vi "Sample Rate Read.vi"(4 "error in (no error)":errorcluster, 6 "Container State":T2, 7 "Display State In":T1) -> (0 "error out":errorcluster, 2 "Value":dbl, 3 "Display State Out":T1)   [LabVIEW 2017, in "Test Signal Configuration.xctl"]
uses:
  <vilib>/addons/_XControls/Function Generator Configuration/Test Signal Configuration.xctl
  <vilib>/_xctls/Container State.ctl
  <vilib>/addons/_XControls/Function Generator Configuration/Controls/State.ctl
  <vilib>/_xctls/XControlSupport.lvlib
panel:
  # "Replace the Value Indicator below with an Indicator of desired type.\nDo not remove this Indicator or the others from the connector pane. \nDo not change the connector pane pattern.\nThe Value Indicator should always be the second terminal from top on the output side in the connector pane."
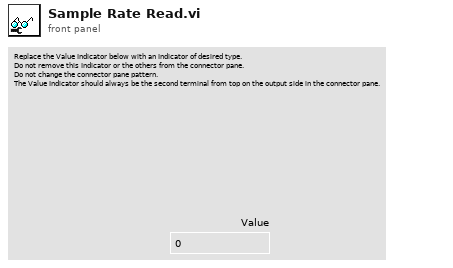
[diagram p1: front panel]
types:
  T1 = typedef "Test Signal Configuration.xctl/State.ctl" = cluster{"Attributes":variant}
  T2 = typedef "XControlSupport.lvlib/Container State.ctl" = cluster{"Indicator?":bool, "Run Mode?":bool, " Refnum":refnum<vi>}
  T3 = typedef "Test Signal Configuration.xctl/signal type.ctl" = enum32{"None", "Tone", "Multitone", "Discrete Sweep", "Continuous Sweep", "Noise"}
  T4 = cluster{"Signal":cluster{"Sample Rate":cluster{"name":string, "default":dbl}, "Signal Type":cluster{"name":string, "signal type":T3}, "Amplitude":cluster{"name":string, "default":dbl}, "Offset":cluster{"name":string, "default":dbl}}, "Function":cluster{"Info":cluster{"name":string, "default":variant}, "Type":cluster{"name":string, "default":u16}, "Frequency":cluster{"name":string, "default":dbl}, "Phase":cluster{"name":string, "default":dbl}}, "Continuous Sweep":cluster{"Info":cluster{"name":string, "default":variant}, "Start":cluster{"name":string, "default":dbl}, "Stop":cluster{"name":string, "default":dbl}, "Duration":cluster{"name":string, "default":dbl}, "Profile":cluster{"name":string, "default":enum16{"Linear", "Logarithmic"}}}, "Discrete Sweep":cluster{"Info":cluster{"name":string, "default":variant}, "Start":cluster{"name":string, "default":dbl}, "Stop":cluster{"name":string, "default":dbl}, "Cycles":cluster{"name":string, "default":dbl}, "Time":cluster{"name":string, "default":dbl}, "Spacing":cluster{"name":string, "default":enum16{"Linear", "Logarithmic"}}, "Steps":cluster{"name":string, "default":i32}}, "Multitone":cluster{"Info":cluster{"name":string, "multitone info":cluster{"frequency":dbl, "amplitude":dbl, "phase":dbl}[]}}, "Noise":cluster{"Info":cluster{"name":string, "default":variant}, "Type":cluster{"name":string, "default":u16}, "Amplitude PDF":cluster{"name":string, "default":enum16{"Gaussian", "Rectangular", "Triangular"}}, "Level":cluster{"name":string, "default":dbl}, "Seed":cluster{"name":string, "default":i32}}, "Configuration":cluster{"Min Frequency":cluster{"name":string, "default":dbl}, "Max Frequency":cluster{"name":string, "default":dbl}, "Max Amplitude":cluster{"name":string, "default":dbl}}}
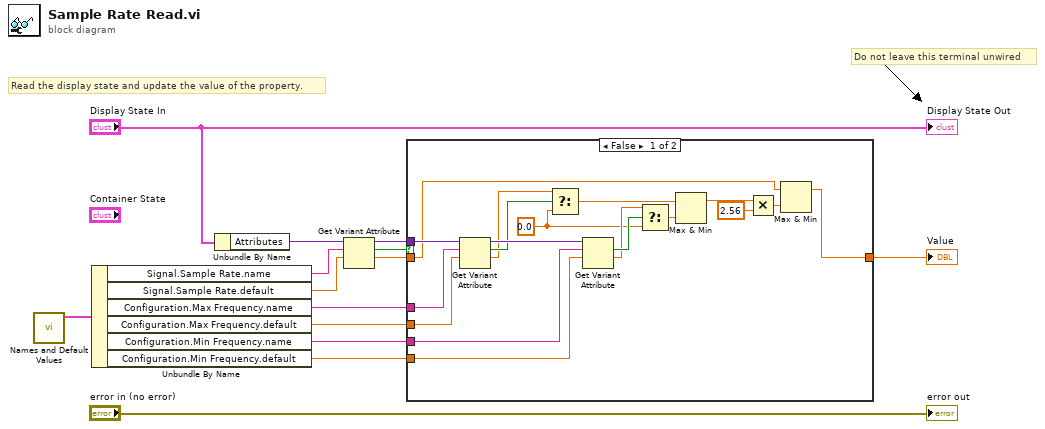
[diagram p0: block diagram]
diagram:
  # "Do not leave this terminal unwired"
  # "Read the display state and update the value of the property."
  n1 = call <vilib>:"Names and Default Values.vi"() -> ("Names and Default Values"=w13:T4)  [unwired: 11 in]
  n2 = Unbundle By Name(w13) -> ("Signal.Sample Rate.name"=w11:string, "Signal.Sample Rate.default"=w9:dbl, "Configuration.Max Frequency.name"=w4:string, "Configuration.Max Frequency.default"=w3:dbl, "Configuration.Min Frequency.name"=w2:string, "Configuration.Min Frequency.default"=w1:dbl)
  n3 = Unbundle By Name("Display State In") -> ("Attributes"=w12:variant)
  n4 = Get Variant Attribute(Variant=w12, name=w11, default value (empty Variant)=w9) -> (duplicate Variant=w5:variant, found=w8:bool, value=w6:dbl)  [unwired: 1 in, 1 out]
  n5 = case shown="False" w8 {
    tunnel: [w15 w33] -> w7
    tunnel: w6 -> [w16 w33]
    tunnel: w5 -> [w32 _]
    tunnel: w4 -> [w31 _]
    tunnel: w3 -> [w30 _]
    tunnel: w2 -> [w28 _]
    tunnel: w1 -> [w27 _]
    frame False {
      w22 = 0.0 ("f")
      n6 = Get Variant Attribute(Variant=w32, name=w31, default value (empty Variant)=w30) -> (duplicate Variant=w29:variant, found=w26:bool, value=w25:dbl)  [unwired: 1 in, 1 out]
      n7 = Select(t=w25, s=w26, f=w22) -> (s? t:f=w21:dbl)
      n8 = Get Variant Attribute(Variant=w29, name=w28, default value (empty Variant)=w27) -> (found=w24:bool, value=w23:dbl)  [unwired: 1 in, 2 out]
      n9 = Select(t=w23, s=w24, f=w22) -> (s? t:f=w20:dbl)
      n10 = Max & Min(x=w21, y=w20) -> (max(x,y)=w19:dbl)  [unwired: 1 out]
      n11 = Multiply(x=w19, y=2.56) -> (x*y=w17:dbl)
      n12 = Max & Min(x=w16, y=w17) -> (max(x,y)=w15:dbl)  [unwired: 1 out]
    }
    frame True {
    }
  }
  "Value" <- w7
  "error out" <- "error in (no error)"
  "Display State Out" <- "Display State In"
